vi "TDMS Write Channel Data.vi"(6 "Fields In":T1[](array[typedef]), 8 "error in (no error)":errorcluster, 9 "Test ID":string, 10 "Test Results":string, 11 "TDMS File Ref":refnum<k34>) -> (0 "error out":errorcluster, 1 "Execution Time (ms)":u32, 3 "TDMS File Ref":refnum<k34>, 4 "Fields Out":T1[](array[typedef]))   [LabVIEW 2011]
uses:
  database/Fields/Field Record.ctl
  database/Fields/Field DataTypes.ctl
  database/Fields/Field NextItem.ctl
  www/tests/Test Function.ctl
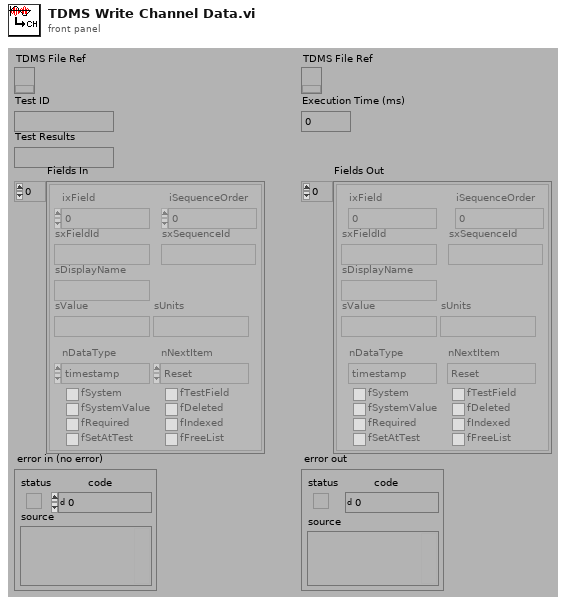
[diagram p1: front panel]
types:
  T1 = typedef "Field Record.ctl" = cluster{"ixField":i32, "iSequenceOrder":i32, "sxFieldId":string, "sxSequenceId":string, "sDisplayName":string, "sValue":string, "sUnits":string, "nDataType":T2, "nNextItem":T3, "fSystem":bool, "fSystemValue":bool, "fRequired":bool, "fSetAtTest":bool, "fTestField":bool, "fDeleted":bool, "fIndexed":bool, "fFreeList":bool}
  T2 = typedef "Field DataTypes.ctl" = enum32{"text", "numeric", "list", "timestamp", "boolean"}
  T3 = typedef "Field NextItem.ctl" = enum32{"Reset", "Retain", "Auto-Increment"}
  T4 = typedef "Test Function.ctl" = enum16{"Test Config", "Test Storage", "Test Pre-Process", "Unflatten Test Parameters", "Flatten Test Parameters"}
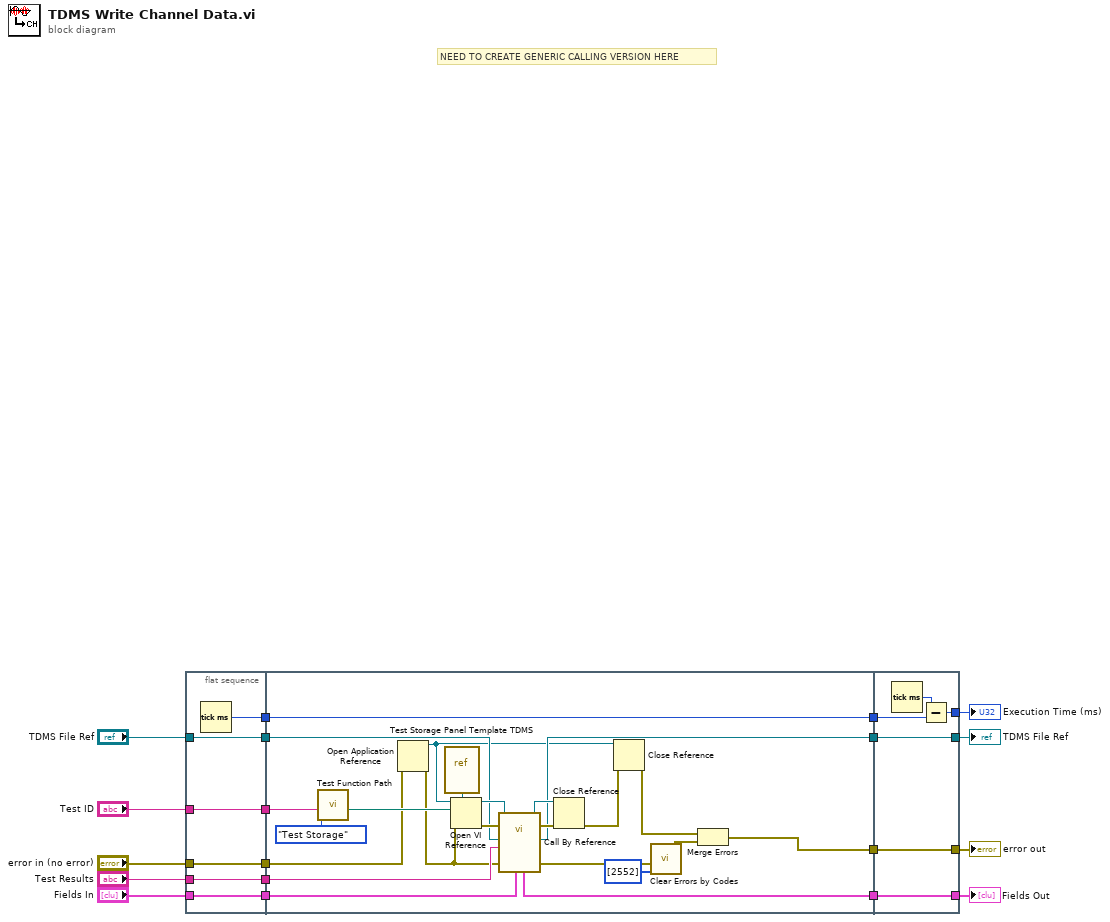
[diagram p0: block diagram]
diagram:
  # "NEED TO CREATE GENERIC CALLING VERSION HERE"
  n1 = flat-sequence {
    tunnel: "TDMS File Ref" -> [w21]
    tunnel: "Test ID" -> [w22]
    tunnel: "Fields In" -> [w23]
    tunnel: "Test Results" -> [w24]
    tunnel: "error in (no error)" -> [w25]
    tunnel: [w25] -> w10
    tunnel: [w24] -> w9
    tunnel: [w23] -> w8
    tunnel: [w22] -> w7
    tunnel: [w21] -> w6
    tunnel: [w20] -> w4
    tunnel: [w42] -> w12
    tunnel: [w36] -> w11
    tunnel: w10 -> [w28]
    tunnel: w9 -> [w40]
    tunnel: w8 -> [w39]
    tunnel: w7 -> [w38]
    tunnel: w6 -> [w37]
    tunnel: [w35] -> w5
    tunnel: w4 -> [w35]
    tunnel: [w31] -> w1
    tunnel: [w53] -> w13
    tunnel: [w54] -> w19
    tunnel: w12 -> [w54]
    tunnel: w11 -> [w53]
    tunnel: w5 -> [w51]
    tunnel: [w50] -> w3
    tunnel: [w49] -> w2
    tunnel: w1 -> [w49]
    frame #0 {
      n2 = Tick Count (ms)() -> (millisecond timer value=w20:u32)
    }
    frame #1 {
      n3 = call "Test Function Path.vi"("Object Type (Test Config)"=Test_Function."Test Storage", "Object Name (\"\")"=w38) -> ("Object Path"=w47:path)  [unwired: 1 in, 8 out]
      n4 = Open Application Reference(8:w28) -> (0:w27:errorcluster, 3:w26:refnum<vi>)  [unwired: 3 in]
      n5 = vi-ref "Test Storage Panel Template TDMS.vi"() -> ("vi reference"=w41:refnum<vi>)
      n6 = Open VI Reference(type specifier VI Refnum (for type only)=w41, application reference (local)=w26, vi path=w47, error in (no error)=w27) -> (vi reference=w46:refnum<vi>, error out=w45:errorcluster)  [unwired: 2 out]
      n7 = call-by-ref "?"(reference=w46, error in=w45, "Fields In"=w39, "error in (no error)"=w27, "Test Results"=w40, "TDMS File Ref"=w37) -> (reference out=w43:refnum<vi>, error out=w44:errorcluster, 0:"error out"=w33:errorcluster, "TDMS File Ref"=w36:refnum<k34>, "Fields Out"=w31:T1[])  [unwired: 5 in]
      n8 = Close Reference(reference=w43, error in (no error)=w44) -> (error out=w30:errorcluster)
      n9 = Close Reference(reference=w26, error in (no error)=w30) -> (error out=w29:errorcluster)
      n10 = call "Clear Errors by Codes.vi"("Error Codes\nto Clear (Empty)"=i32[] [2552] ("Error Codes\nto Clear (Empty)"), "error in (no error)"=w33) -> ("error out"=w32:errorcluster)  [unwired: 5 out]
      n11 = Merge Errors(w29, w32) -> (w42:errorcluster)
    }
    frame #2 {
      n12 = Tick Count (ms)() -> (millisecond timer value=w52:u32)
      n13 = Subtract(x=w52, y=w51) -> (x-y=w50:u32)
    }
  }
  "error out" <- w19
  "TDMS File Ref" <- w13
  "Execution Time (ms)" <- w3
  "Fields Out" <- w2
